vi "write_samples_per_sec.vi"(0 "Byte Stream File in":T1, 1 "task in":refnum<k21>, 2 "Volume":dbl(slide) scale=0.0..0.5, 3 "Playback speed":dbl(knob) scale=0.25..2.0, 5 "Sample offset":u64, 9 "Samples per channel":dbl, 11 "error in":errorcluster) -> (4 "Refnum out":refnum<k21>, 6 "next_offset":u64, 8 "data out":waveform(dbl), 10 "end of file?":bool, 15 "error out":errorcluster)   [LabVIEW 2022 SP3]
uses:
  <vilib>/sound2/lvsound2.llb/Sound File Refnum.ctl
  <vilib>/sound2/lvsound2.llb/Sound File Position.ctl
  <vilib>/DAQmx/miscellaneous.llb/DAQmx Fill In Error Info.vi
  <vilib>/sound2/lvsound2.llb/Sound File Read (DBL).vi
  <vilib>/DAQmx/write.llb/DAQmx Write (Analog Wfm 1Chan NSamp).vi
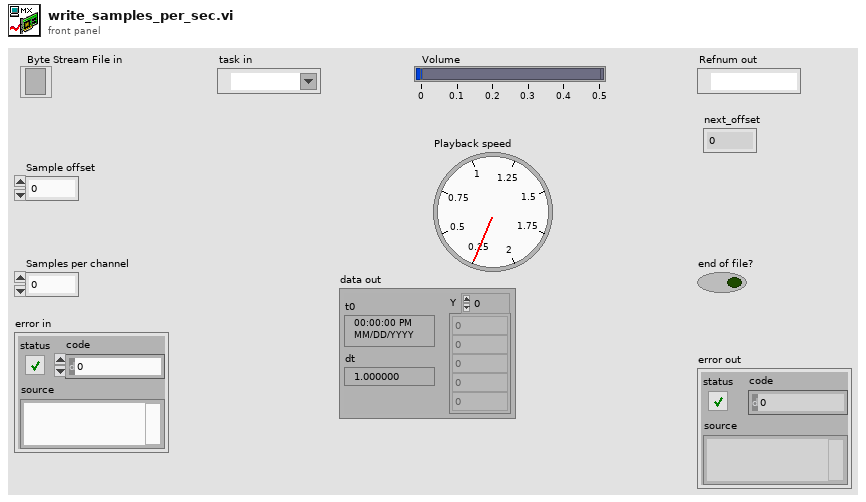
[diagram p1: front panel]
types:
  T1 = typedef "Sound File Refnum.ctl" = refnum<file>
  T2 = typedef "Sound File Position.ctl" = u16
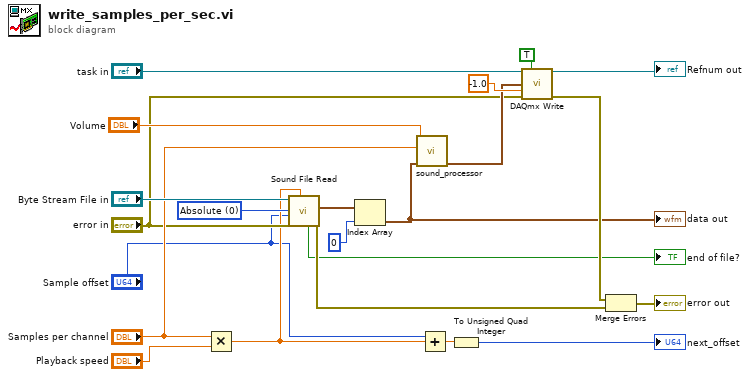
[diagram p0: block diagram]
diagram:
  w11 = T2 0 items=["Absolute"=0, "Relative"=2] ("position mode")
  n1 = Multiply(x="Samples per channel", y="Playback speed") -> (x*y=w4:dbl)
  n2 = call-poly <vilib>:"Sound File Read.vi"("number of samples/ch (-1: all)"=w4, "error in (no error)"="error in", "position offset"="Sample offset", "position mode"=w11, "sound file refnum"="Byte Stream File in") -> ("error out"=w14:errorcluster, "data"=w16:waveform(dbl)[], "end of file?"=→"end of file?":bool)  [unwired: 2 in, 2 out]
  n3 = Index Array(array=w16, index=0) -> (element=w5:waveform(dbl))
  "data out" <- w5
  n4 = call "sound_processor.vi"("data in"=w5, "Target samples per channel"="Samples per channel", "Volume"="Volume") -> ("data out"=w8:waveform(dbl))  [unwired: 8 in]
  n5 = Add(x="Sample offset", y=w4) -> (x+y=w2:dbl)
  n6 = To Unsigned Quad Integer(1:w2) -> (0:→"next_offset":u64)
  n7 = call-poly <vilib>:"DAQmx Write.vi"("task/channels in"="task in", "auto start"=TRUE, "data"=w8, "timeout"=-1.0, "error in"="error in") -> ("task out"=→"Refnum out":refnum<k21>, "error out"=w18:errorcluster)  [unwired: 8 in, 1 out]
  n8 = Merge Errors(w18, w14) -> (→"error out":errorcluster)
